vi "Fetch Multi Eval Meas PSD Trace Results.vi"(8 "error in (no error)":errorcluster, 9 "Result Type (Current)":i32(ring) items=["Current"=0, "Average"=1, "Maximum"=4], 10 "Instance (1)":i32=1, 11 "VISA resource name":refnum<visa-resource-name>) -> (0 "error out":errorcluster, 1 "Results":dbl[](array[numeric]) format="%^.3e", 2 "Reliability":i32, 3 "VISA resource name out":refnum<visa-resource-name>)   [LabVIEW 2020, in "Rohde&Schwarz CMP LR WPAN Measurement.lvlib"]
doc: "Returns the power spectral density traces measured using a 100 kHz resolution bandwidth filter. The results are relative to the maximum average spectral power measured within the 1.0 MHz of the carrier frequency. The first and last samples correspond to -12.5 MHz and +12.5 MHz relative to the carrier frequency. The frequency step between two consecutive samples is 31.25 kHz.\n\nAttribute:\n-\n\nRemote-control commands:\nFETCh:WPAN:MEAS<i>:MEValuation:TRACe:PSDensity:CURRent[:RELative]?\nFETCh:WPAN:MEAS<i>:MEValuation:TRACe:PSDensity:AVERage[:RELative]?\nFETCh:WPAN:MEAS<i>:MEValuation:TRACe:PSDensity:MAXimum[:RELative]?"
uses:
  <instrlib>/Rohde&Schwarz CMP LR WPAN Measurement/Rohde&Schwarz CMP LR WPAN Measurement.lvlib
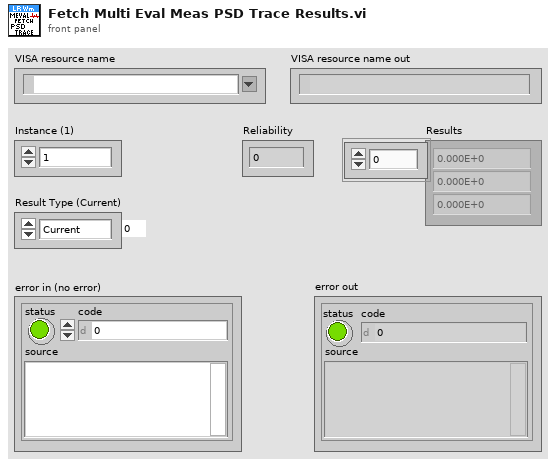
[diagram p1: front panel]
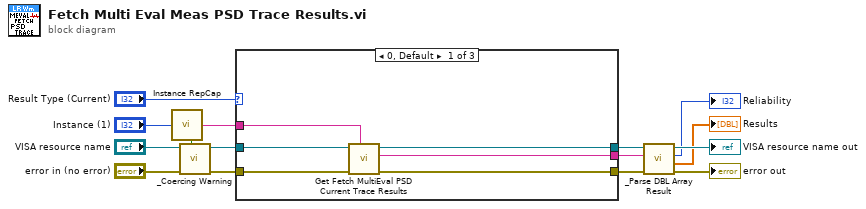
[diagram p0: block diagram]
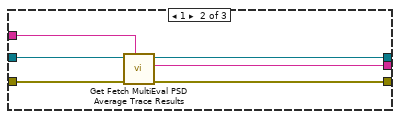
[diagram p2: hidden frame]
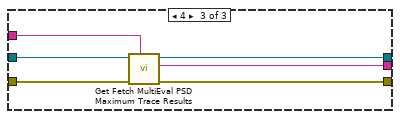
[diagram p3: hidden frame]
diagram:
  n1 = call <instrlib>:"Instance RepCap.vi"("Instance In"="Instance (1)") -> ("In Range?"=w12:bool, "RepCap Identifier Out"=w15:string)  [unwired: 1 in]
  n2 = call <instrlib>:"_Coercing Warning.vi"("In Range?"=w12, "error in (no error)"="error in (no error)", "VISA resource name"="VISA resource name") -> ("error out"=w14:errorcluster, "VISA resource name out"=w13:refnum<visa-resource-name>)  [unwired: 7 in]
  n3 = case shown="0, Default" "Result Type (Current)" {
    tunnel: w15 -> [w21 w27 w31]
    tunnel: w13 -> [w20 w26 w32]
    tunnel: w14 -> [w19 w25 w33]
    tunnel: [w18 w24 w30] -> w7
    tunnel: [w17 w23 w29] -> w8
    tunnel: [w16 w22 w28] -> w4
    frame 0, Default {
      n4 = call "Get Fetch MultiEval PSD Current Trace Results"("Repeated Capabilities"=w21, "error in (no error)"=w19, "instrument handle"=w20) -> ("error out"=w17:errorcluster, "Fetch MultiEval PSD Current Trace Results"=w16:string, "instrument handle out"=w18:refnum<visa-resource-name>)  [unwired: 6 in]
    }
    frame 1 {
      n5 = call "Get Fetch MultiEval PSD Average Trace Results"("Repeated Capabilities"=w27, "error in (no error)"=w25, "instrument handle"=w26) -> ("error out"=w23:errorcluster, "Fetch MultiEval PSD Average Trace Results"=w22:string, "instrument handle out"=w24:refnum<visa-resource-name>)  [unwired: 6 in]
    }
    frame 4 {
      n6 = call "Get Fetch MultiEval PSD Maximum Trace Results"("Repeated Capabilities"=w31, "error in (no error)"=w33, "instrument handle"=w32) -> ("error out"=w29:errorcluster, "Fetch MultiEval PSD Maximum Trace Results"=w28:string, "instrument handle out"=w30:refnum<visa-resource-name>)  [unwired: 6 in]
    }
  }
  n7 = call <instrlib>:"_Parse DBL Array Result.vi"("error in (no error)"=w8, "Input String"=w4, "VISA resource name"=w7) -> ("error out"=→"error out":errorcluster, "Results"=→"Results":dbl[], "Reliability"=→"Reliability":i32, "VISA resource name out"=→"VISA resource name out":refnum<visa-resource-name>)  [unwired: 5 in]
